vi "Assert Client Id.vi"(8 "expected unique id":u64, 9 "actual unique id":u64, 10 "expected client id":u64, 11 "actual client id":u64) -> (2 "result":string, 3 "pass":bool)   [LabVIEW 2020, in "MeasurementServerTests.lvlib" / "Discovery Tests.lvlib"]
uses:
  Discovery Tests.lvlib
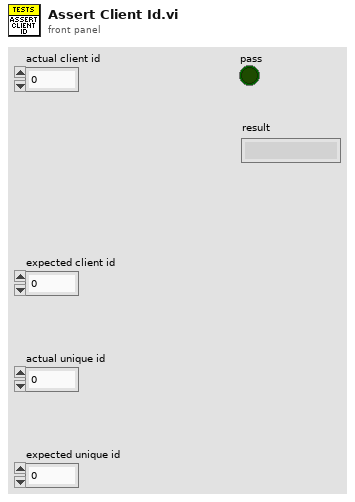
[diagram p1: front panel]
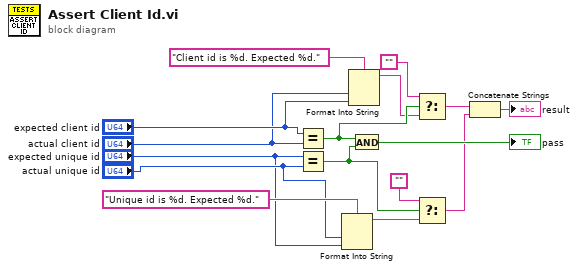
[diagram p0: block diagram]
diagram:
  n1 = Equal?(x="expected client id", y="actual client id") -> (x = y?=w13:bool)
  n2 = Equal?(x="expected unique id", y="actual unique id") -> (x = y?=w7:bool)
  n3 = Format Into String(format string="Unique id is %d. Expected %d.", "actual unique id", "expected unique id") -> (resulting string=w6:string)  [unwired: 2 in, 1 out]
  n4 = Format Into String(format string="Client id is %d. Expected %d.", "actual client id", "expected client id") -> (resulting string=w12:string)  [unwired: 2 in, 1 out]
  n5 = And(x=w13, y=w7) -> (x .and. y?=→"pass":bool)
  n6 = Select(t="", s=w13, f=w12) -> (s? t:f=w11:string)
  n7 = Select(t="", s=w7, f=w6) -> (s? t:f=w3:string)
  n8 = Concatenate Strings(w11, w3) -> (→"result":string)
